vi "CNN_probe.vi"(11 "CNN out":refnum<class "CNN.lvclass">) -> (2 "Value String":string, 3 "Boolean":bool)   [LabVIEW 2016, in "CNN.lvclass"]
uses:
  CNN.lvclass
  CNN.lvclass/CNN.ctl
panel:
  out "Firing rate":cluster{i32, dbl, dbl[]}[](graph)
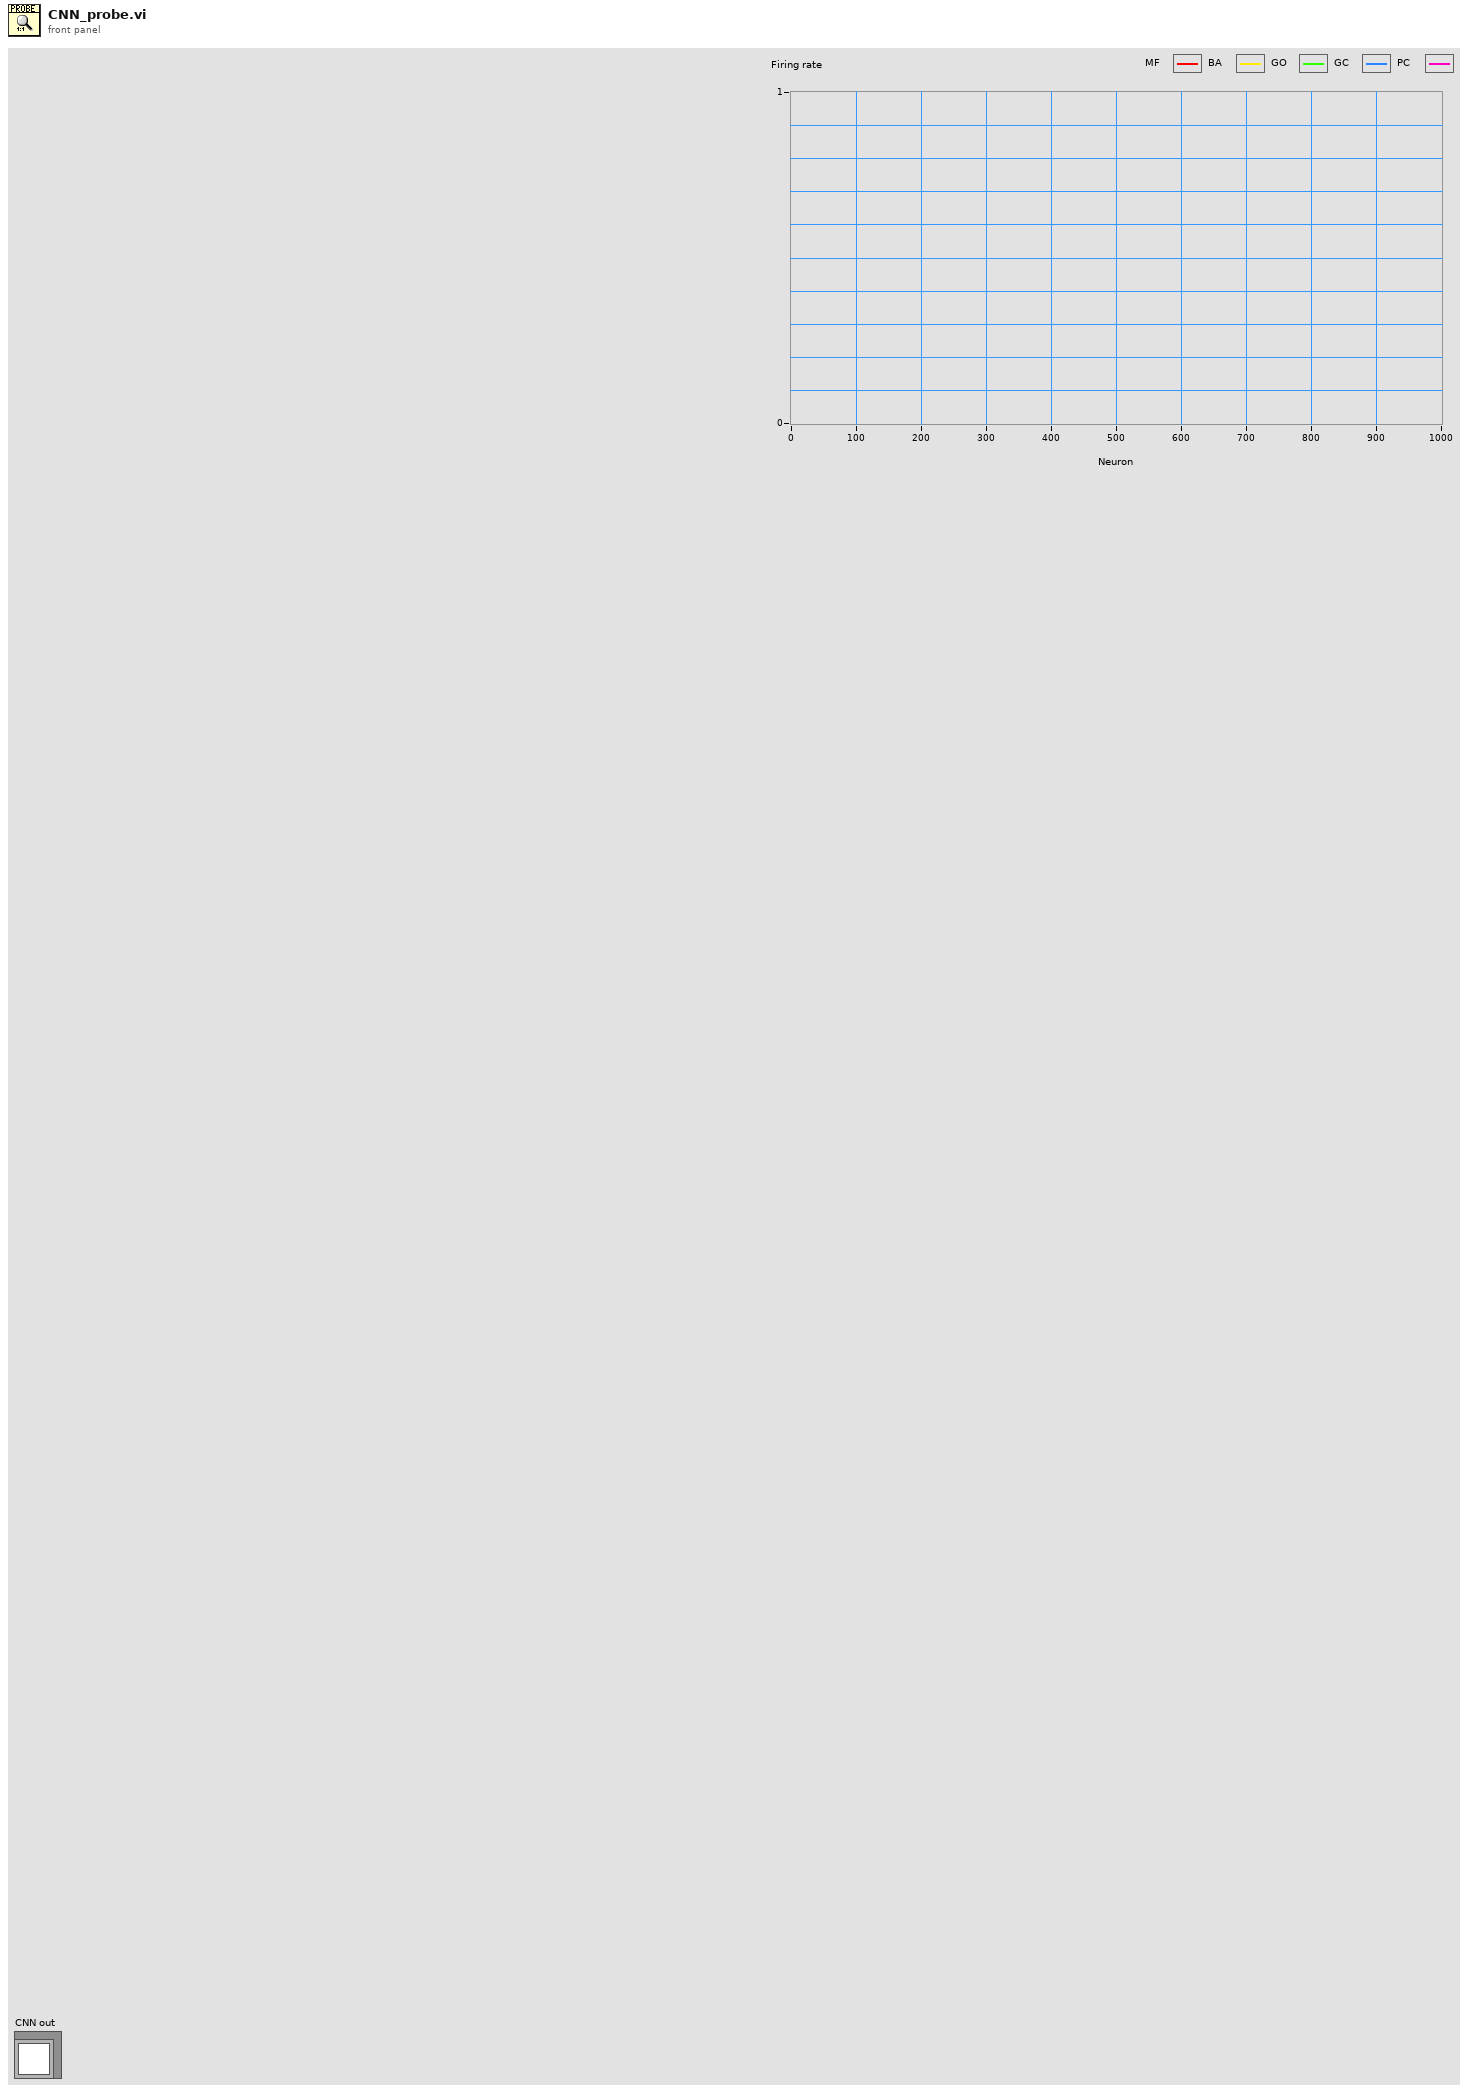
[diagram p1: front panel]
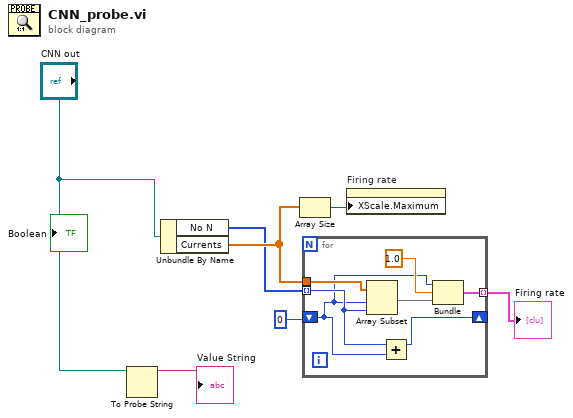
[diagram p0: block diagram]
diagram:
  n1 = To Probe String(7:"CNN out") -> (3:→"Value String":string)  [unwired: 2 in, 1 out]
  n2 = Unbundle By Name("CNN out") -> ("No N"=w2:i32[], "Currents"=w3:dbl[])
  n3 = Array Size(array=w3) -> (size(s)=w4:i32)
  n4 = for {
    tunnel: w2 -> [w13] mode=indexing
    tunnel: w3 -> [w14]
    shift-right: [w9] -> _
    shift-left: 0 -> [w8]
    tunnel: [w10] -> w5 mode=indexing
    n5 = Array Subset(array=w14, index=w8, length=w13) -> (w12:dbl[])
    n6 = Add(x=w13, y=w8) -> (x+y=w9:i32)
    n7 = Bundle(w8, 1.0, w12) -> (w10:cluster{i32, dbl, dbl[]})  [unwired: 1 in]
  }
  "Firing rate" <- w5
  n8 = property on="Firing rate" class="WFGraph (strict)"("XScale.Maximum"=w4) -> ()  [unwired: 2 in, 2 out]
